vi "Update Measurement Selection.vi"(8 "error in (no error)":errorcluster, 10 "mouseDown coords":T1, 11 "multicolumnListbox in":refnum<vi>) -> (0 "error out":errorcluster, 3 "multicolumnListbox out":refnum<vi>)   [LabVIEW 2021, in "MeasurementClient Editor.lvlib"]
uses:
  MeasurementClient Editor.lvlib
  <vilib>/Utility/miscctls.llb/LVPoint32TypeDef.ctl
  <vilib>/Utility/miscctls.llb/LVPositionTypeDef.ctl
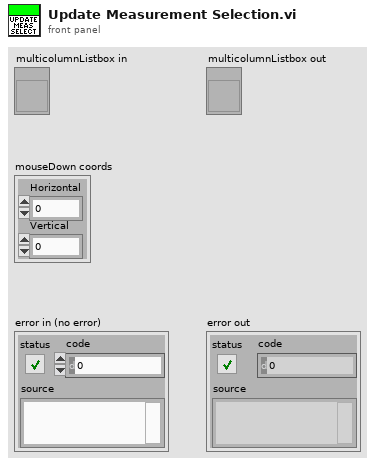
[diagram p1: front panel]
types:
  T1 = typedef "LVPoint32TypeDef.ctl" = cluster{"Horizontal":i32, "Vertical":i32}
  T2 = typedef "LVPositionTypeDef.ctl" = cluster{"Left":i32, "Top":i32}
  T3 = typedef "LVRowAndColumnTypeDef.ctl" = cluster{"Row":i32, "Column":i32}
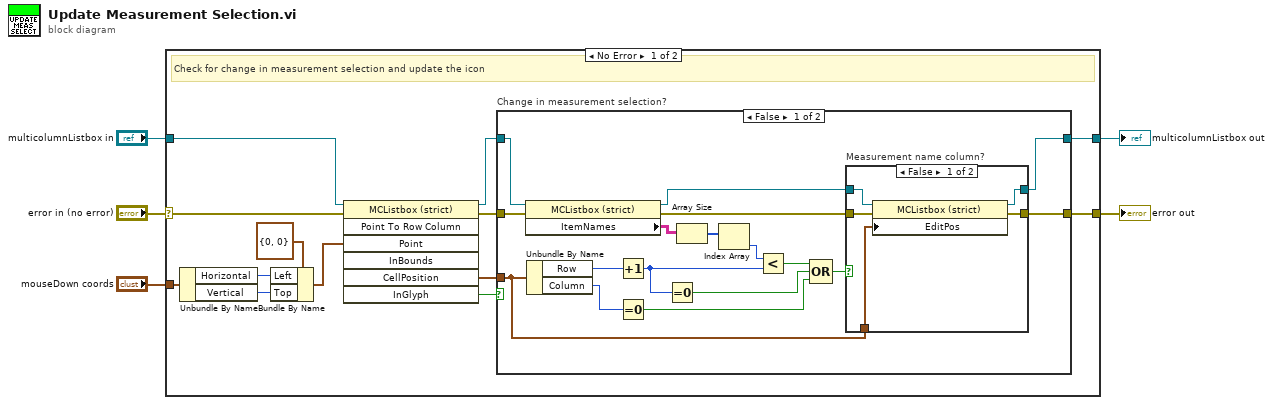
[diagram p0: block diagram]
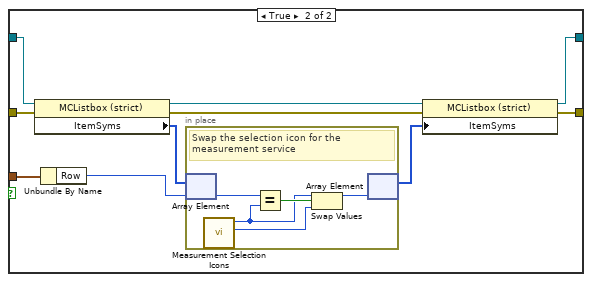
[diagram p3: hidden frame]
diagram:
  n1 = case shown="No Error" "error in (no error)" {
    selector: "error in (no error)" -> [w13 w58]
    tunnel: [w18 w58] -> w5
    tunnel: [w7 w59] -> w4
    tunnel: "multicolumnListbox in" -> [w14 w59]
    tunnel: "mouseDown coords" -> [w12 _]
    frame No Error {
      # "Check for change in measurement selection and update the icon"
      n2 = Unbundle By Name(w12) -> ("Horizontal"=w9:i32, "Vertical"=w8:i32)
      n3 = Bundle By Name(cluster=T2 {"Left"=0, "Top"=0} ("Point"), "Left"=w9, "Top"=w8) -> (w10:T2)
      n4 = invoke class="MCListbox (strict)" method="Point To Row Column"(reference=w14, error in=w13, "Point"=w10) -> (reference out=w17:refnum<vi>, error out=w15:errorcluster, "CellPosition"=w16:T3, "InGlyph"=w6:bool)  [unwired: 4 in, 3 out]
      n5 = case "Change in measurement selection?" shown="False" w6 {
        tunnel: w15 -> [w28 w52]
        tunnel: w16 -> [w24 w50]
        tunnel: w17 -> [w27 w51]
        tunnel: [w26 w47] -> w7
        tunnel: [w25 w46] -> w18
        frame False {
          n6 = property class="MCListbox (strict)"(reference=w27, error in=w28) -> (reference out=w29:refnum<vi>, error out=w34:errorcluster, "ItemNames"=w33:string[][])
          n7 = Unbundle By Name(w24) -> ("Row"=w30:i32, "Column"=w35:i32)
          n8 = Increment(x=w30) -> (x+1=w23:i32)
          n9 = Equal To 0?(x=w35) -> (x = 0?=w21:bool)
          n10 = Equal To 0?(x=w23) -> (x = 0?=w22:bool)
          n11 = Array Size(array=w33) -> (size(s)=w32:i32[])
          n12 = Index Array(array=w32) -> (element=w31:i32)  [unwired: 1 in]
          n13 = Less?(x=w31, y=w23) -> (x < y?=w20:bool)
          n14 = Compound Arithmetic op=OR(w20, w22, w21) -> (w19:bool)
          n15 = case "Measurement name column?" shown="False" w19 {
            tunnel: w34 -> [w40 w42]
            tunnel: [w39 w42] -> w25
            tunnel: [w38 w41] -> w26
            tunnel: w29 -> [w37 w41]
            tunnel: w24 -> [w36 _]
            frame False {
              n16 = property class="MCListbox (strict)"(reference=w37, error in=w40, "EditPos"=w36) -> (reference out=w38:refnum<vi>, error out=w39:errorcluster)
            }
            frame True {
            }
          }
        }
        frame True {
          n17 = property class="MCListbox (strict)"(reference=w51, error in=w52) -> (reference out=w49:refnum<vi>, error out=w48:errorcluster, "ItemSyms"=w45:i32[])
          n18 = Unbundle By Name(w50) -> ("Row"=w43:i32)
          n19 = in-place {
            # "Swap the selection icon for the measurement service"
            n20 = in-place-array #1(w45, w43) -> (w57:i32)
            n21 = call "Measurement Selection Icons.vi"() -> ("Checked"=w53:i32, "Unchecked"=w54:i32)  [unwired: 10 in]
            n22 = Equal?(x=w57, y=w54) -> (x = y?=w55:bool)
            n23 = Swap Values(12:w54, 13:w55, 14:w53) -> (1:w56:i32)  [unwired: 1 out]
            n24 = in-place-array #1(w56) -> (w44:i32[])  [unwired: 1 out]
          }
          n25 = property class="MCListbox (strict)"(reference=w49, error in=w48, "ItemSyms"=w44) -> (reference out=w47:refnum<vi>, error out=w46:errorcluster)
        }
      }
    }
    frame Error {
      # "Pass"
    }
  }
  "error out" <- w5
  "multicolumnListbox out" <- w4
